vi "DMM_Scan PMPS 16V-15C Initialize.vi"(0 "Scan Resources Names":T2={"DMM Resource Name"="DMM_4080", "MUX Resource Name"="MUX_2527", "Shunt Resource Name"="Shunt_2568"}, 2 "Powerline Frequency":T7=enum."50 Hz", 5 "Topology":T5={"MUX Topology Name"="2527/2-Wire Dual 16x1 Mux", "Shunt Topology Name"="2568/31-SPST"}, 7 "Close all Shunts?":bool=TRUE, 11 "error in":errorcluster) -> (4 "Scan Resource Handles Out":T1 caption="Scan Resource Handles out", 6 "Switches Characteristics":T3, 15 "error out":errorcluster)   [LabVIEW 2021, in "DMM_Scan PXI Mux PXI Shunt 16V-15C.lvlib"]
doc: "Creates a new NI-DMM Scan driver session on each device specified in the Scan Resource Names control configured with the local powerline frequency. The devices use the powerline frequency value to select a timebase for setting the Aperture Time property in powerline cycles (PLCs). Change the Powerline Frequency value to 60 Hz for North & South America.\n\nA specific switch topology associated to a fixed channel mapping is defined by default for the random 16 voltage and 15 current configuration. Each channel number for current is linked to the same channel shunt number. (ex. Current ch16 = Shunt ch16)\n\nThe \"Close all Shunts\" input control is used to close all relays from channels 16 to 30 (NI 2568) in a fixed channel topology mapping, allowing continuous power to the DUT during all measurements. Deselect \"Close all shunts\" to open current shunts. For example, deselect \"Close all shunts\" in the instance of a 2-Wire Resistance measurement function without any current through the DUT.\n\nThe VI returns the max voltage and current characteristics from each multiplexer and shunt relay."
uses:
  DMM_Scan PXI Mux PXI Shunt 16V-15C.lvlib
  <instrlib>/niDMM/nidmm.llb/niDMM Powerline Frequency.ctl
  Typedefs/Topology.ctl
  <instrlib>/niSwitch/niSwitch.llb/niSwitch Topologies.ctl
  Typedefs/Switches Characteristics.ctl
  Static Digital Path Generation/Typedefs/Module Characteristics.ctl
  Typedefs/Scan Resource Names.ctl
  Typedefs/Scan Resource Handles Out.ctl
  Static Digital Path Generation/Typedefs/Terminal and State Settings.ctl
  DMM Mixed Measurements/DMM_Mixed Measurement.lvlib
  Static Digital Path Generation/Switch_Static Digital Path Generation.lvlib
panel:
  # "Inputs"
  # "Outputs"
  # "Overview:\nThis VI interacts with the NI-DMM and NI-SWITCH drivers to initialize NI-DMM instruments and provide a corresponding instrument handle according to the topology selected\n\nHardware Requirements: A PXI, PCIe, or USB DMM instrument, any switch with the same topology as NI-2527 MUX and NI-2568 Relay\n\nSoftware Requirements: NI-DMM 2022 Q3 or above, NI-SWITCH 2022 Q4 or above\n\nInstructions:\nSelect your DMM instrument resource name in the drop down control\nSelect your Multiplexer Switch resource\nSelect your Current Shunt Relay resource\nSelect each topology (In the configuration 16 voltage + 15 current, default values are \"2527/2-Wire Dual 16x1 Mux\" and \"2568/31-SPST\"\n\nNote: each \"DMM Handle Out\" indicator will be used by the Configure & Measure and Close API functions"
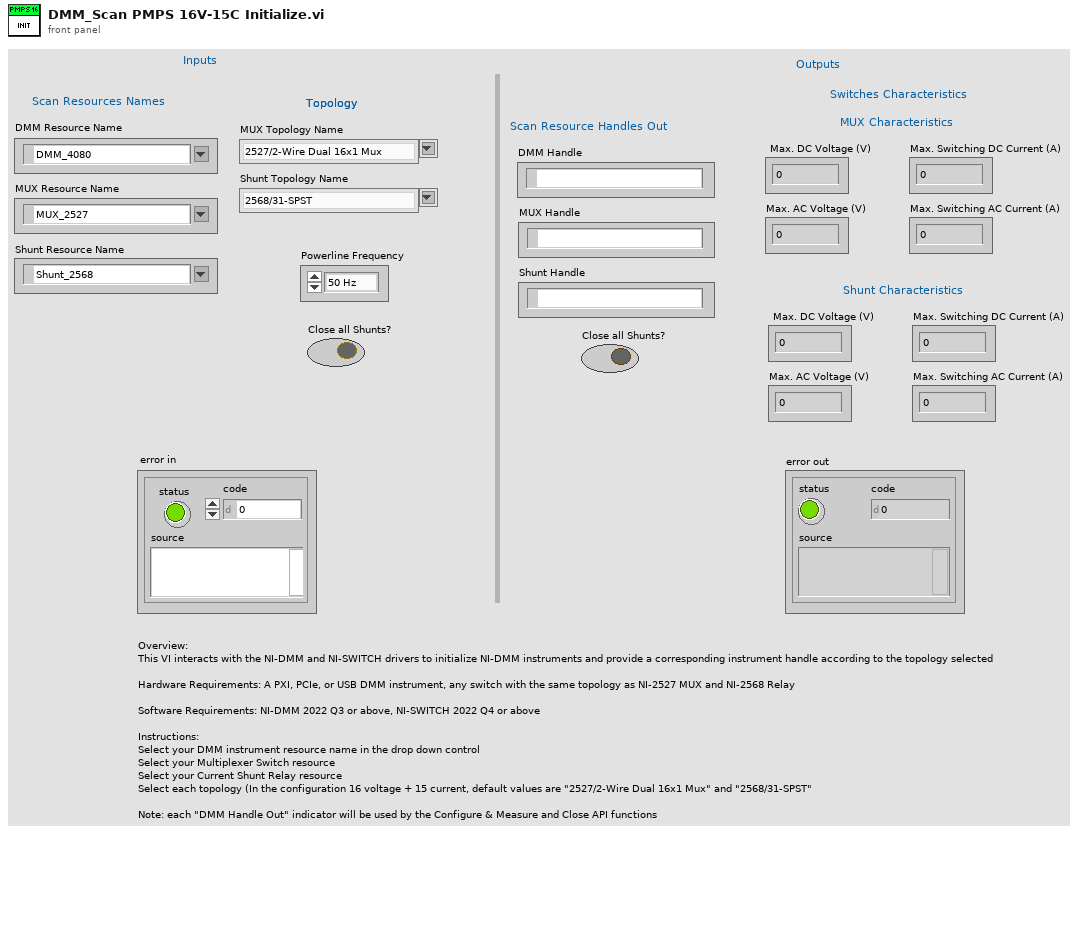
[diagram p1: front panel]
types:
  T1 = typedef "DMM_Scan PXI Mux PXI Shunt 16V-15C.lvlib/Scan Resource Handles Out.ctl" = cluster{"DMM Handle":refnum<k15>, "MUX Handle":refnum<k15>, "Shunt Handle":refnum<k15>, "Close all Shunts?":bool}
  T2 = typedef "DMM_Scan PXI Mux PXI Shunt 16V-15C.lvlib/Scan Resource Names.ctl" = cluster{"DMM Resource Name":refnum<k15>, "MUX Resource Name":refnum<k15>, "Shunt Resource Name":refnum<k15>}
  T3 = typedef "DMM_Scan PXI Mux PXI Shunt 16V-15C.lvlib/Switches Characteristics.ctl" = cluster{"Mux Characteristics":T4, "Shunt Characteristics":T4}
  T4 = typedef "Switch_Static Digital Path Generation.lvlib/Module Characteristics.ctl" = cluster{" Max. DC Voltage (V)":dbl, "Max. Switching DC Current (A)":dbl, "Max. AC Voltage (V)":dbl, "Max. Switching AC Current (A)":dbl}
  T5 = typedef "DMM_Scan PXI Mux PXI Shunt 16V-15C.lvlib/Topology.ctl" = cluster{"MUX Topology Name":T6, "Shunt Topology Name":T6}
  T6 = typedef "niSwitch Topologies.ctl" = string
  T7 = typedef "niDMM Powerline Frequency.ctl" = enum16{"60 Hz", "50 Hz"}
  T8 = typedef "Switch_Static Digital Path Generation.lvlib/Terminal and State Settings.ctl" = cluster{"Connect/Disconnect":bool, "Channel 1":string, "Channel 2":string}
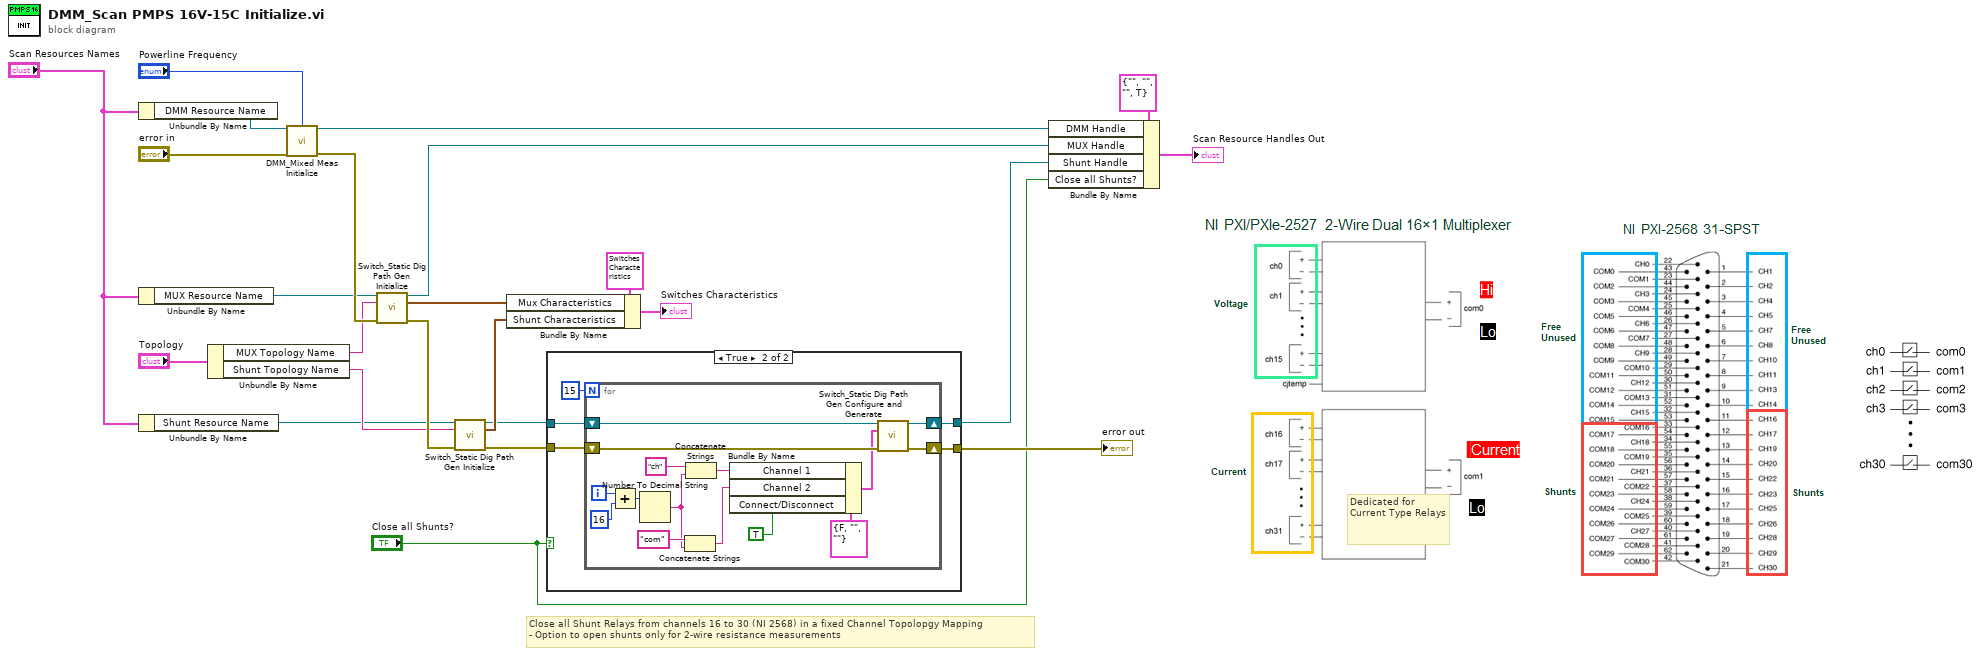
[diagram p0: block diagram]
diagram:
  # "Dedicated for Current Type Relays"
  # "Close all Shunt Relays from channels 16 to 30 (NI 2568) in a fixed Channel Topolopgy Mapping\n- Option to open shunts only for 2-wire resistance measurements"
  n1 = Unbundle By Name("Scan Resources Names") -> ("DMM Resource Name"=w13:refnum<k15>)
  n2 = Unbundle By Name("Scan Resources Names") -> ("MUX Resource Name"=w12:refnum<k15>)
  n3 = Unbundle By Name("Scan Resources Names") -> ("Shunt Resource Name"=w11:refnum<k15>)
  n4 = Unbundle By Name("Topology") -> ("MUX Topology Name"=w20:T6, "Shunt Topology Name"=w18:T6)
  n5 = call "DMM_Mixed Meas Initialize.vi"("DMM Resource Name"=w13, "Powerline Frequency"="Powerline Frequency", "error in"="error in") -> ("DMM Handle Out"=w10:refnum<k15>, "error out"=w24:errorcluster)  [unwired: 11 in]
  n6 = call "Switch_Static Dig Path Gen Initialize.vi"("Switch Resource Name"=w12, "Topology Name"=w20, "error in"=w24) -> ("Switch Handle Out"=w9:refnum<k15>, "Module Characteristics"=w17:T4, "error out"=w22:errorcluster)  [unwired: 10 in]
  n7 = call "Switch_Static Dig Path Gen Initialize.vi"("Switch Resource Name"=w11, "Topology Name"=w18, "error in"=w22) -> ("Switch Handle Out"=w6:refnum<k15>, "Module Characteristics"=w16:T4, "error out"=w5:errorcluster)  [unwired: 10 in]
  n8 = Bundle By Name(cluster=T3 {"Mux Characteristics"={" Max. DC Voltage (V)"=300.0, "Max. Switching DC Current (A)"=2.0, "Max. AC Voltage (V)"=300.0, "Max. Switching AC Current (A)"=2.0}, "Shunt Characteristics"={" Max. DC Voltage (V)"=150.0, "Max. Switching DC Current (A)"=2.0, "Max. AC Voltage (V)"=150.0, "Max. Switching AC Current (A)"=2.0}} ("Switches Characteristics"), "Mux Characteristics"=w17, "Shunt Characteristics"=w16) -> (→"Switches Characteristics":T3)
  n9 = case shown="True" "Close all Shunts?" {
    tunnel: w6 -> [w26 w31]
    tunnel: [w26 w30] -> w3
    tunnel: w5 -> [w25 w29]
    tunnel: [w25 w28] -> w4
    frame False {
    }
    frame True {
      n10 = for {
        N: 15 -> [_]
        shift-right: [w45] -> w30
        shift-left: w31 -> [w46]
        shift-right: [w43] -> w28
        shift-left: w29 -> [w44]
        i -> [w42]
        n11 = Add(x=w42, y=16) -> (x+y=w40:i32)
        n12 = Number To Decimal String(number=w40) -> (decimal integer string=w33:string)  [unwired: 1 in]
        n13 = Concatenate Strings("com" ("string"), w33) -> (w32:string)
        n14 = Concatenate Strings("ch" ("string"), w33) -> (w35:string)
        n15 = Bundle By Name(cluster=T8 {"Connect/Disconnect"=FALSE, "Channel 1"="", "Channel 2"=""} ("Terminal and State Settings"), "Channel 1"=w35, "Channel 2"=w32, "Connect/Disconnect"=TRUE) -> (w39:T8)
        n16 = call "Switch_Static Dig Path Gen Configure and Generate.vi"("Switch Handle In"=w46, "Terminal and State Settings"=w39, "error in"=w44) -> ("Switch Handle Out"=w45:refnum<k15>, "error out"=w43:errorcluster)  [unwired: 10 in, 1 out]
      }
    }
  }
  "error out" <- w4
  n17 = Bundle By Name(cluster=T1 {"DMM Handle"="", "MUX Handle"="", "Shunt Handle"="", "Close all Shunts?"=TRUE} ("Scan Handles Out"), "DMM Handle"=w10, "MUX Handle"=w9, "Shunt Handle"=w3, "Close all Shunts?"="Close all Shunts?") -> (→"Scan Resource Handles Out":T1)
